vi "ask position from stages.vi"(8 "error in (no error)":errorcluster, 11 "Autofocus in":refnum<class "Autofocus.lvclass">) -> (0 "error out":errorcluster, 3 "Autofocus out":refnum<class "Autofocus.lvclass">)   [LabVIEW 2012, in "Autofocus.lvclass"]
uses:
  Autofocus.lvclass
  <vilib>/Distrio/Murmex/GenericMessage/GenericMessage.lvclass
  Autofocus.lvclass/Autofocus.ctl
  <vilib>/Distrio/Murmex/Message/Add or replace parameter.vi
  <vilib>/Distrio/Murmex/Murmex/Murmex.lvclass
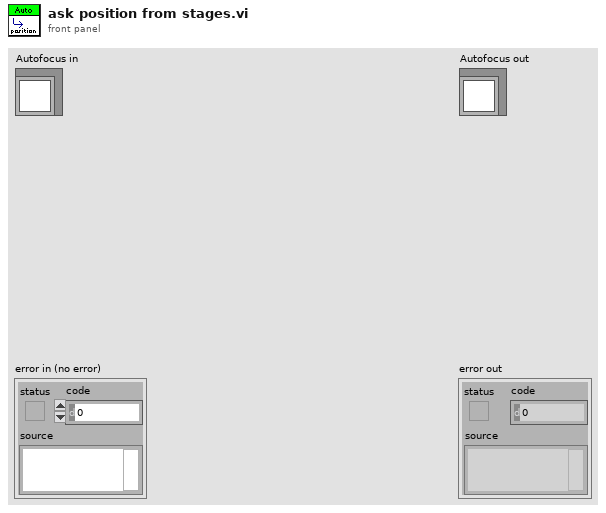
[diagram p1: front panel]
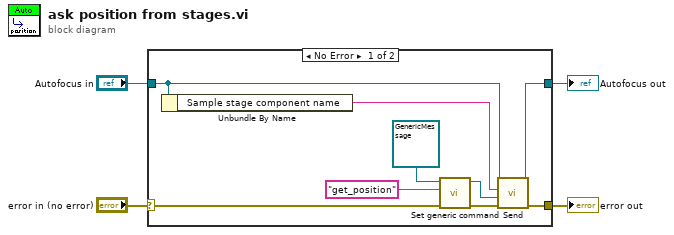
[diagram p0: block diagram]
diagram:
  n1 = case shown="No Error" "error in (no error)" {
    selector: "error in (no error)" -> [w13 w15]
    tunnel: [w9 w15] -> w3
    tunnel: [w7 w14] -> w1
    tunnel: "Autofocus in" -> [w6 w14]
    frame No Error {
      n2 = Unbundle By Name(w6) -> ("Sample stage component name"=w5:string)
      n3 = call <vilib>:"Set generic command.vi"("error in (no error)"=w13, "generic command"="get_position", "GenericMessage in"=refnum<class "GenericMessage.lvclass"> refnum ("Message in")) -> ("error out"=w10:errorcluster, "GenericMessage out"=w8:refnum<class "GenericMessage.lvclass">)  [unwired: 7 in]
      n4 = call <vilib>:"Send.vi"("error in (no error)"=w10, "Message"=w8, "recipient"=w5, "Murmex in"=w6) -> ("error out"=w9:errorcluster, "Murmex out"=w7:refnum<class "Autofocus.lvclass">)  [unwired: 6 in]
    }
    frame Error {
    }
  }
  "error out" <- w3
  "Autofocus out" <- w1
